vi "ExDataCollectFocus1Strip.vi"() -> ()   [LabVIEW 2010]
uses:
  Open-Close Hardware/CamHandle.vi
panel:
  out "Strip":u16[](graph)
  in  "Stop collection":bool
  out "ready to \nstart":bool
  in  "Start collection":bool
  in  "Exposure":dbl=0.004 min=0.0 step=0.001 format="%.3f"
  out "error out":errorcluster
  in  "error in (no error)":errorcluster
  # "ExDataCollectFocus1Strip:\nthis example collects data for 1 strips.\nRun this vi and wait for the ready to start to turn green.\nThen hit the start button to collect and display the strip as graph"
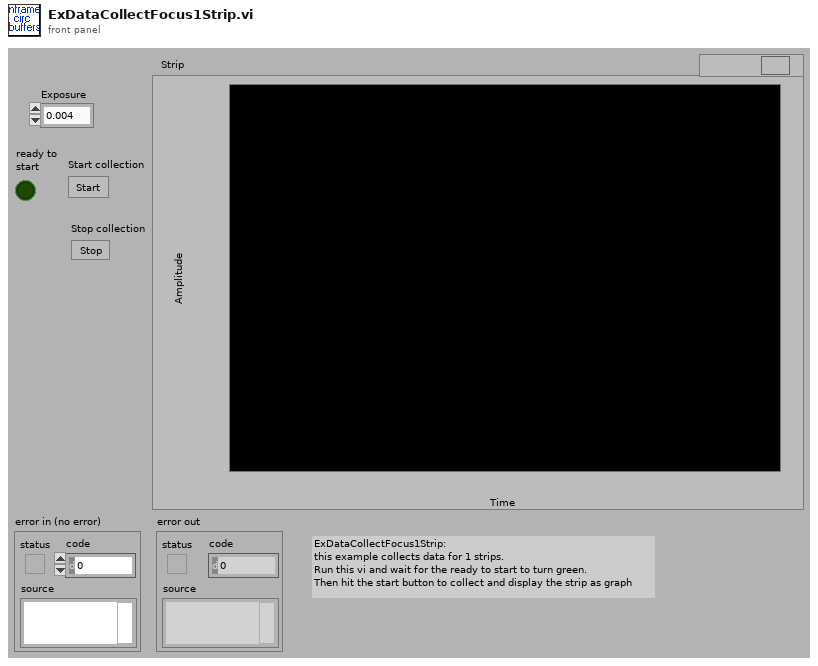
[diagram p1: front panel]
types:
  T1 = cluster{"acquire focus mode":u32, "Exposure":dbl, i32, "Software accumulation":u32}
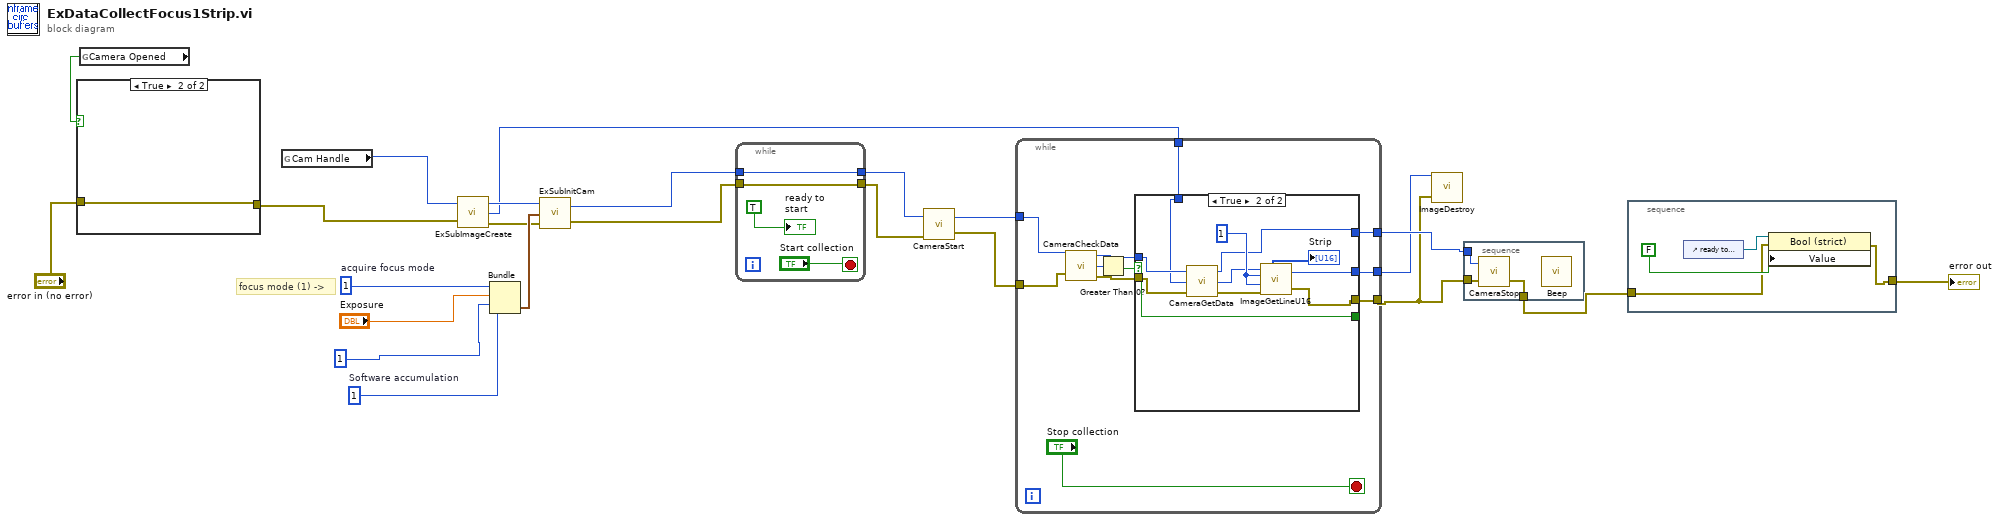
[diagram p0: block diagram]
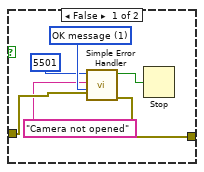
[diagram p3: hidden frame]
diagram:
  w21 = u32 1  # acquire focus mode
  w20 = u32 1  # Software accumulation
  # "focus mode (1) ->"
  n1 = global read "CamHandle.vi" "Camera Opened"() -> (w18:bool)
  n2 = case shown="True" w18 {
    tunnel: "error in (no error)" -> [w28 w30]
    tunnel: [w27 w30] -> w12
    frame False {
      w29 = u16 1 items=["no dialog", "OK message", "continue or stop message"] ("type of dialog (OK msg:1)")
      n3 = call <vilib>:"Simple Error Handler.vi"("error code (no error:0)"=5501, "error source (\" \")"="Camera not opened", "type of dialog (OK msg:1)"=w29, "error in (no error)"=w28) -> ("error?"=w25:bool, "error out"=w27:errorcluster)  [unwired: 1 in, 3 out]
      n4 = Stop(stop? (T)=w25) -> ()
    }
    frame True {
    }
  }
  n5 = global read "CamHandle.vi" "Cam Handle"() -> (w14:u32)
  n6 = call "ExSubImageCreate.vi"("Camera Handle"=w14, "error in (no error)"=w12) -> ("Camera Handle"=w13:u32, "Data Handle"=w10:u32, "error out"=w11:errorcluster)
  n7 = Bundle("acquire focus mode"=w21, "Exposure"="Exposure", 1, "Software accumulation"=w20) -> (w22:T1)  [unwired: 1 in]
  n8 = call "ExSubInitCam.vi"("error in (no error)"=w11, "Camera Information"=w22, "Camera Handle"=w13) -> ("error out"=w4:errorcluster, "Camera Handle"=w2:u32)
  n9 = while {
    tunnel: w4 -> [w32]
    tunnel: [w32] -> w3
    tunnel: w2 -> [w31]
    tunnel: [w31] -> w1
    stop <- "Start collection" stop-if-true
    "ready to \nstart" <- TRUE
  }
  n10 = call <userlib>:"CameraStart.vi"("error in"=w3, "Camera Handle"=w1) -> ("error out"=w15:errorcluster, "Camera Handle"=w16:u32)
  n11 = while {
    tunnel: w16 -> [w41]
    tunnel: w15 -> [w40]
    tunnel: w10 -> [w38]
    tunnel: [w37] -> w7
    tunnel: [w36] -> w6
    tunnel: [w35] -> w9
    stop <- "Stop collection" stop-if-true
    n12 = call <userlib>:"CameraCheckData.vi"("Camera Handle"=w41, "error in"=w40) -> ("Camera Handle"=w43:u32, "Number Of Frames Available"=w45:i32, "error out"=w42:errorcluster)
    n13 = Greater Than 0?(x=w45) -> (x > 0?=w44:bool)
    n14 = case shown="True" w44 {
      selector: w44 -> [w48 w58]
      tunnel: w43 -> [w46 w60]
      tunnel: w42 -> [w49 w59]
      tunnel: [w48 w58] -> _
      tunnel: [w49 w56] -> w36
      tunnel: w38 -> [w47 w55]
      tunnel: [w47 w53] -> w37
      tunnel: [w46 w52] -> w35
      frame False {
      }
      frame True {
        w54 = 1
        n15 = call <userlib>:"CameraGetData.vi"("error in"=w59, "Data Handle"=w55, "Camera Handle"=w60) -> ("error out"=w51:errorcluster, "Data Handle"=w50:u32, "Camera Handle"=w52:u32)
        n16 = call <userlib>:"ImageGetLineU16.vi"("Data Handle"=w50, "Y Position"=w54, "Z Position"=w54, "error in"=w51) -> ("Array u16"=→"Strip":u16[], "Data Handle"=w53:u32, "error out"=w56:errorcluster)
      }
    }
  }
  n17 = call <userlib>:"ImageDestroy.vi"("error in"=w6, "Data handle"=w7) -> ()  [unwired: 1 out]
  n18 = stacked-sequence {
    tunnel: w9 -> [w63]
    tunnel: [w62] -> w8
    tunnel: w6 -> [w61]
    frame #0 {
      n19 = call <userlib>:"CameraStop.vi"("error in"=w61, "Camera Handle"=w63) -> ("error out"=w62:errorcluster)  [unwired: 1 out]
      n20 = call <vilib>:"Beep.vi"() -> ()  [unwired: 12 in]
    }
  }
  n21 = stacked-sequence {
    tunnel: [w65] -> w17
    tunnel: w8 -> [w64]
    frame #0 {
      n22 = control-ref of="ready to \nstart"() -> (w67:refnum<vi>)
      n23 = property class="Bool (strict)"(reference=w67, error in=w64, "Value"=FALSE) -> (error out=w65:errorcluster)  [unwired: 1 out]
    }
  }
  "error out" <- w17
